vi "GetVIPaths.vi"(4 "MenuType":T1, 5 "error in (no error)":errorcluster) -> (0 "error out":errorcluster, 2 "SubMenu VIs":path[](array[path]), 3 "Menu VIs":path[](array[path]))   [LabVIEW 2023]
uses:
  MenuType.ctl
panel:
  # "Output"
  # "Input"
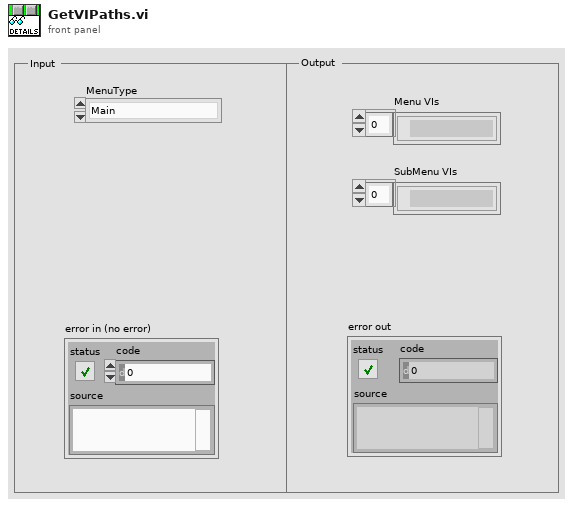
[diagram p1: front panel]
types:
  T1 = typedef "MenuType.ctl" = enum16{"Main", "Simulation", "ME", "SF", "User Utilities", "Dev Tools"}
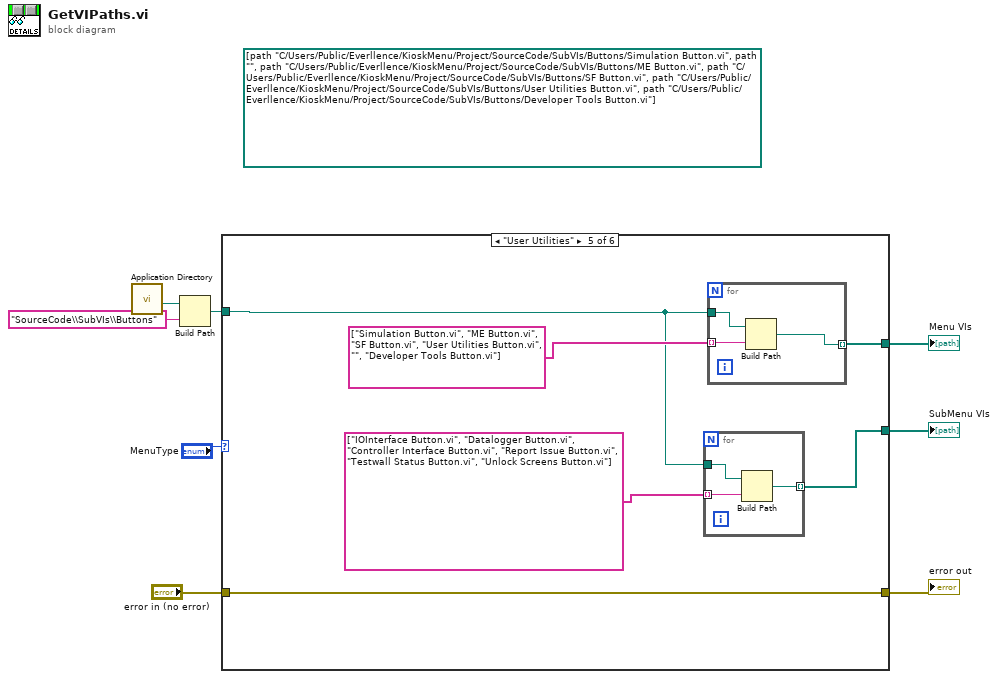
[diagram p0: block diagram]
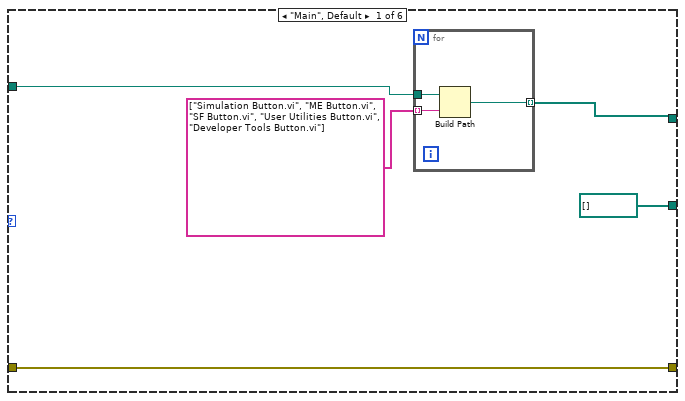
[diagram p2: hidden frame]
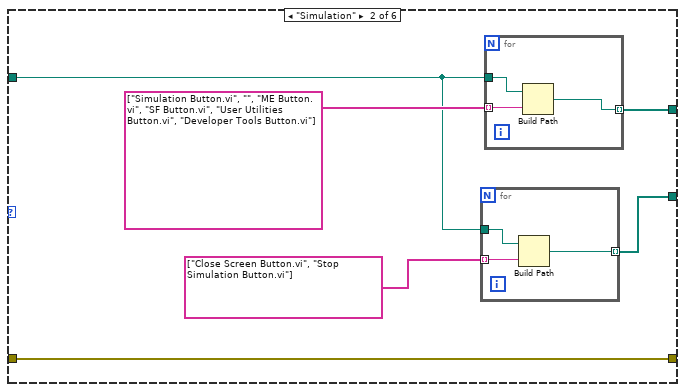
[diagram p3: hidden frame]
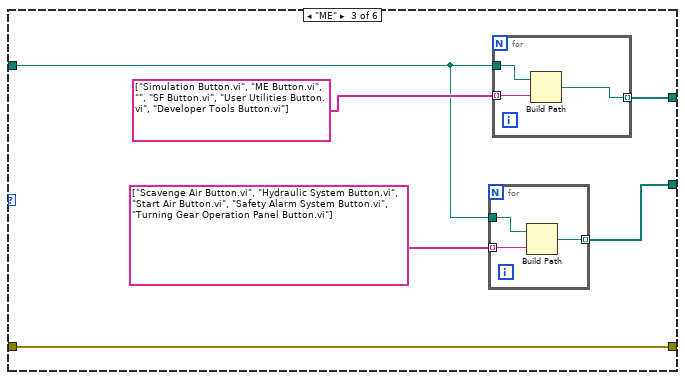
[diagram p4: hidden frame]
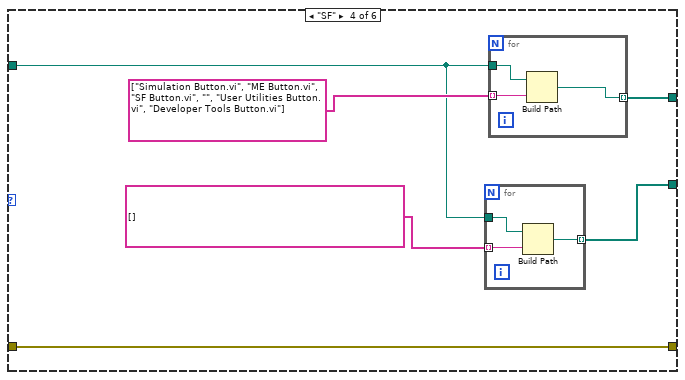
[diagram p5: hidden frame]
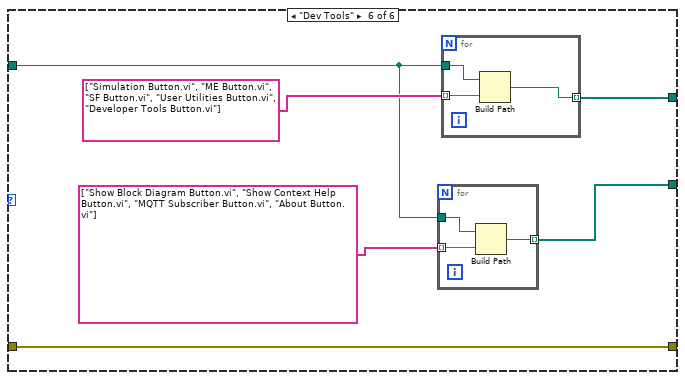
[diagram p6: hidden frame]
diagram:
  (unwired) path[] [path "C:/Users/Public/Everllence/KioskMenu/Project/SourceCode/SubVIs/Buttons/Simulation Button.vi", path "", path "C:/Users/Public/Everllence/KioskMenu/Project/SourceCode/SubVIs/Buttons/ME Button.vi", path "C:/Users/Public/Everllence/KioskMenu/Project/SourceCode/SubVIs/Buttons/SF Button.vi", path "C:/Users/Public/Everllence/KioskMenu/Project/SourceCode/SubVIs/Buttons/User Utilities Button.vi", path "C:/Users/Public/Everllence/KioskMenu/Project/SourceCode/SubVIs/Buttons/Developer Tools Button.vi"]
  n1 = call <vilib>:"Application Directory.vi"() -> ("Application Directory"=w3:path)
  n2 = Build Path(base path=w3, name or relative path="SourceCode\\SubVIs\\Buttons") -> (appended path=w1:path)
  n3 = case shown="\"User Utilities\"" "MenuType" {
    tunnel: [w10 w20 w30 w42 w54 w65] -> w8
    tunnel: "error in (no error)" -> [w13 w22 w34 w46 w58 w70]
    tunnel: [w13 w22 w34 w46 w58 w70] -> w5
    tunnel: [path[] [] ("SubMenu VIs") w19 w29 w41 w53 w66] -> w4
    tunnel: w1 -> [w9 w18 w31 w43 w55 w67]
    frame "Main", Default {
      n4 = for {
        tunnel: string[] ["Simulation Button.vi", "ME Button.vi", "SF Button.vi", "User Utilities Button.vi", "Developer Tools Button.vi"] -> [w16] mode=indexing
        tunnel: [w15] -> w10 mode=indexing
        tunnel: w9 -> [w14]
        n5 = Build Path(base path=w14, name or relative path=w16) -> (appended path=w15:path)
      }
    }
    frame "Simulation" {
      n6 = for {
        tunnel: w18 -> [w25]
        tunnel: string[] ["Close Screen Button.vi", "Stop Simulation Button.vi"] -> [w24] mode=indexing
        tunnel: [w23] -> w19 mode=indexing
        n7 = Build Path(base path=w25, name or relative path=w24) -> (appended path=w23:path)
      }
      n8 = for {
        tunnel: w18 -> [w28]
        tunnel: string[] ["Simulation Button.vi", "", "ME Button.vi", "SF Button.vi", "User Utilities Button.vi", "Developer Tools Button.vi"] -> [w27] mode=indexing
        tunnel: [w26] -> w20 mode=indexing
        n9 = Build Path(base path=w28, name or relative path=w27) -> (appended path=w26:path)
      }
    }
    frame "ME" {
      n10 = for {
        tunnel: w31 -> [w37]
        tunnel: string[] ["Scavenge Air Button.vi", "Hydraulic System Button.vi", "Start Air Button.vi", "Safety Alarm System Button.vi", "Turning Gear Operation Panel Button.vi"] -> [w36] mode=indexing
        tunnel: [w35] -> w29 mode=indexing
        n11 = Build Path(base path=w37, name or relative path=w36) -> (appended path=w35:path)
      }
      n12 = for {
        tunnel: w31 -> [w40]
        tunnel: string[] ["Simulation Button.vi", "ME Button.vi", "", "SF Button.vi", "User Utilities Button.vi", "Developer Tools Button.vi"] -> [w39] mode=indexing
        tunnel: [w38] -> w30 mode=indexing
        n13 = Build Path(base path=w40, name or relative path=w39) -> (appended path=w38:path)
      }
    }
    frame "SF" {
      n14 = for {
        tunnel: w43 -> [w49]
        tunnel: string[] [] -> [w48] mode=indexing
        tunnel: [w47] -> w41 mode=indexing
        n15 = Build Path(base path=w49, name or relative path=w48) -> (appended path=w47:path)
      }
      n16 = for {
        tunnel: w43 -> [w52]
        tunnel: string[] ["Simulation Button.vi", "ME Button.vi", "SF Button.vi", "", "User Utilities Button.vi", "Developer Tools Button.vi"] -> [w51] mode=indexing
        tunnel: [w50] -> w42 mode=indexing
        n17 = Build Path(base path=w52, name or relative path=w51) -> (appended path=w50:path)
      }
    }
    frame "User Utilities" {
      n18 = for {
        tunnel: w55 -> [w61]
        tunnel: string[] ["IOInterface Button.vi", "Datalogger Button.vi", "Controller Interface Button.vi", "Report Issue Button.vi", "Testwall Status Button.vi", "Unlock Screens Button.vi"] -> [w60] mode=indexing
        tunnel: [w59] -> w53 mode=indexing
        n19 = Build Path(base path=w61, name or relative path=w60) -> (appended path=w59:path)
      }
      n20 = for {
        tunnel: w55 -> [w64]
        tunnel: string[] ["Simulation Button.vi", "ME Button.vi", "SF Button.vi", "User Utilities Button.vi", "", "Developer Tools Button.vi"] -> [w63] mode=indexing
        tunnel: [w62] -> w54 mode=indexing
        n21 = Build Path(base path=w64, name or relative path=w63) -> (appended path=w62:path)
      }
    }
    frame "Dev Tools" {
      n22 = for {
        tunnel: w67 -> [w73]
        tunnel: string[] ["Show Block Diagram Button.vi", "Show Context Help Button.vi", "MQTT Subscriber Button.vi", "About Button.vi"] -> [w72] mode=indexing
        tunnel: [w71] -> w66 mode=indexing
        n23 = Build Path(base path=w73, name or relative path=w72) -> (appended path=w71:path)
      }
      n24 = for {
        tunnel: w67 -> [w76]
        tunnel: string[] ["Simulation Button.vi", "ME Button.vi", "SF Button.vi", "User Utilities Button.vi", "Developer Tools Button.vi"] -> [w75] mode=indexing
        tunnel: [w74] -> w65 mode=indexing
        n25 = Build Path(base path=w76, name or relative path=w75) -> (appended path=w74:path)
      }
    }
  }
  "error out" <- w5
  "Menu VIs" <- w8
  "SubMenu VIs" <- w4
